vi "Generate CRC-16.vi"(7 "DATA PACKET":string) -> (1 "CRC-16 value":u16 format="%x", 2 "RCR-16 bytes":u8[](array[numeric]) format="%x", 3 "CRC-16 H-str":string)   [LabVIEW 2021, in "F-70 driver.lvlib"]
doc: "Calculates CRC-16 for messages to/from F-70 compressor (maximum 64 characters) and outputs it as string of its hexadecimal representation. Optionaly, an uint_8 array or direct uint_16 value can be outputed.\n\nDerived from example VI found at: forums.ni.com/t5/Example-Code/CRC-16-Calculator/ta-p/3996194"
uses:
  <instrlib>/F-70 driver/F-70 driver.lvlib
panel:
  # "Example: \nMessage \"$ID1\" will have checksum 0xD629\nString that needs to be send via RS-232 is: \"$ID1D629\\r\""
  # "The checksum is a 16 bit CRC. It is transmitted as four-digit ASCII hex.\nExample: a 16 bit binary checksum “001001110101011” in four-digit\nASCII equals \"23AB\". The check sum calculation includes the “$” start\ncharacter, command field, data fields (if present), and all commas\nincluding the comma preceding the checksum. See section E below for\ndescription of CRC-16 generation.\n\n\n\nCRC-16 ANSI (also MODBUS) is used. The CRC-16 is first started by pre-loading a 16 bit\nregister with all 1's. The process begins by applying successive 8-bit bytes of the message\nto the current contents of the register. Only the eight bits of the data in each character are\nused for generating the CRC. Start, stop, and parity bits do not apply to the CRC.\nDuring generation of the CRC, each 8-bit character is Exclusive-ORed (XORed) with the\nregister contents. Then the result is shifted in the direction of the least significant bit (LSB),\nwith a zero filling the most significant bit (MSB). The LSB is then examined. If the LSB is a\n1, the register is XORed with a preset fixed value (A001h). If the LSB is a 0, then no XOR\ntakes place.\nThis process is repeated until eight shifts have been performed. After the last shift, then the\nnext 8-bit message byte is XORed with the 16-bit register. The eight-shift processes above\nare repeated.\nAfter all of the message bytes have been XORed and shifted, the result is the CRC."
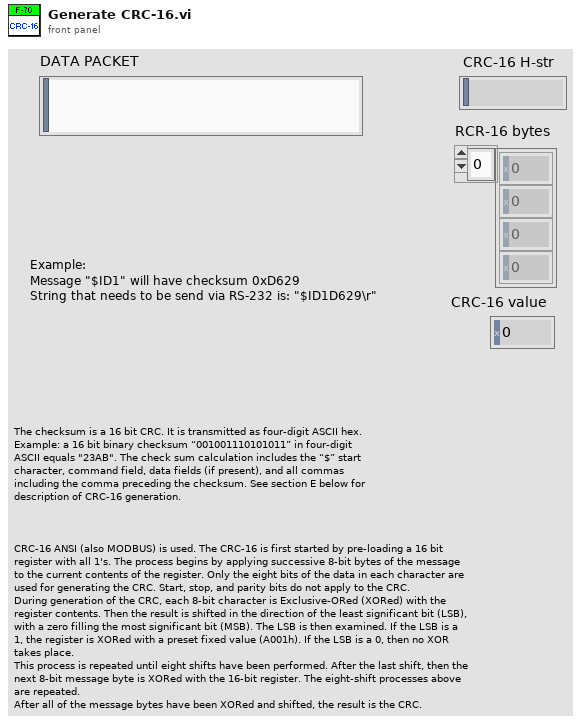
[diagram p1: front panel]
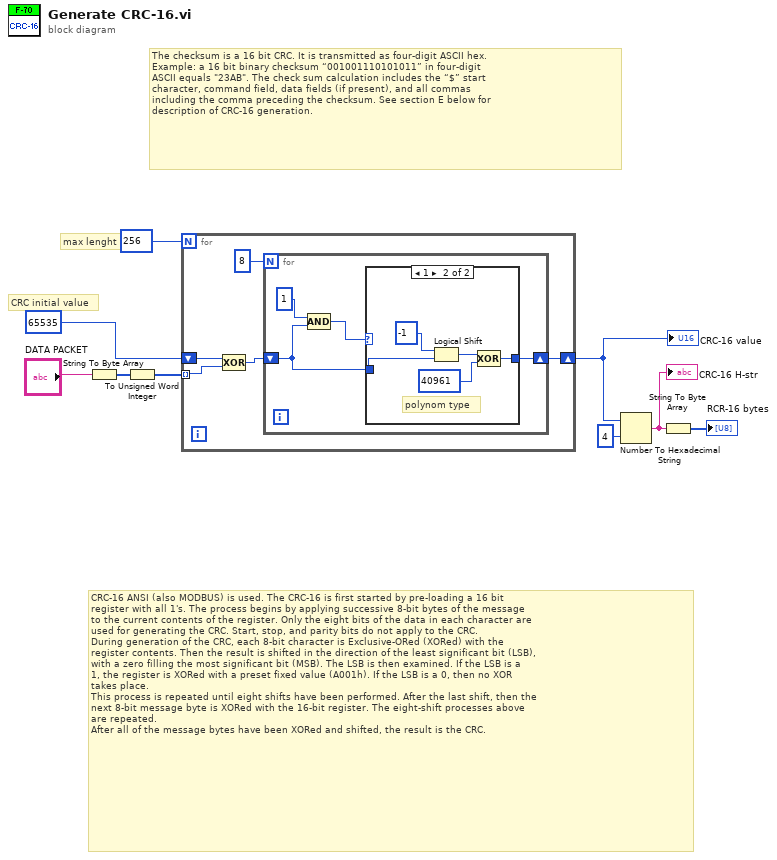
[diagram p0: block diagram]
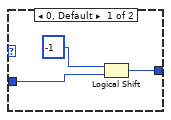
[diagram p2: hidden frame]
diagram:
  # "CRC-16 ANSI (also MODBUS) is used. The CRC-16 is first started by pre-loading a 16 bit\nregister with all 1's. The process begins by applying successive 8-bit bytes of the message\nto the current contents of the register. Only the eight bits of the data in each character are\nused for generating the CRC. Start, stop, and parity bits do not apply to the CRC.\nDuring generation of the CRC, each 8-bit character is Exclusive-ORed (XORed) with the\nregister contents. Then the result is shifted in the direction of the least significant bit (LSB),\nwith a zero filling the most significant bit (MSB). The LSB is then examined. If the LSB is a\n1, the register is XORed with a preset fixed value (A001h). If the LSB is a 0, then no XOR\ntakes place.\nThis process is repeated until eight shifts have been performed. After the last shift, then the\nnext 8-bit message byte is XORed with the 16-bit register. The eight-shift processes above\nare repeated.\nAfter all of the message bytes have been XORed and shifted, the result is the CRC."
  # "The checksum is a 16 bit CRC. It is transmitted as four-digit ASCII hex.\nExample: a 16 bit binary checksum “001001110101011” in four-digit\nASCII equals \"23AB\". The check sum calculation includes the “$” start\ncharacter, command field, data fields (if present), and all commas\nincluding the comma preceding the checksum. See section E below for\ndescription of CRC-16 generation."
  # "max lenght"
  # "CRC initial value"
  n1 = String To Byte Array(string="DATA PACKET") -> (unsigned byte array=w6:u8[])
  n2 = To Unsigned Word Integer(number=w6) -> (unsigned 16bit integer=w5:u16[])
  n3 = for {
    N: 256 ("Numeric") -> [_]
    shift-right: [w11] -> w4
    shift-left: u16 65535 -> [w12]
    tunnel: w5 -> [w10] mode=indexing
    n4 = Compound Arithmetic op=XOR(w12, w10) -> (w13:u32)
    n5 = for {
      N: 8 -> [_]
      shift-right: [w17] -> w11
      shift-left: w13 -> [w16]
      n6 = Compound Arithmetic op=AND(u16 1, w16) -> (w15:u32)
      n7 = case shown="1" w15 {
        tunnel: [w20 w25] -> w17
        tunnel: w16 -> [w19 w22]
        frame 0, Default {
          n8 = Logical Shift(y=i16 -1, x=w19) -> (x << y=w20:u32)
        }
        frame 1 {
          # "polynom type"
          n9 = Logical Shift(y=i16 -1, x=w22) -> (x << y=w24:u32)
          n10 = Compound Arithmetic op=XOR(w24, u32 40961) -> (w25:u32)
        }
      }
    }
  }
  "CRC-16 value" <- w4
  n11 = Number To Hexadecimal String(1:i16 4 ("width (-)"), 2:w4) -> (0:w2:string)
  "CRC-16 H-str" <- w2
  n12 = String To Byte Array(string=w2) -> (unsigned byte array=→"RCR-16 bytes":u8[])
